vi "get_resolution.vi"(8 "error in (no error)":errorcluster, 11 "TrajectoryDL090201FrameScan in":refnum<class "TrajectoryDL090201FrameScan.lvclass">) -> (0 "error out":errorcluster, 1 "y":i32, 2 "x":i32, 3 "TrajectoryDL090201FrameScan out":refnum<class "TrajectoryDL090201FrameScan.lvclass">)   [LabVIEW 2010, in "TrajectoryDL090201FrameScan.lvclass"]
uses:
  TrajectoryDL090201FrameScan.lvclass
  TrajectoryDL090201FrameScan.lvclass/TrajectoryDL090201FrameScan.ctl
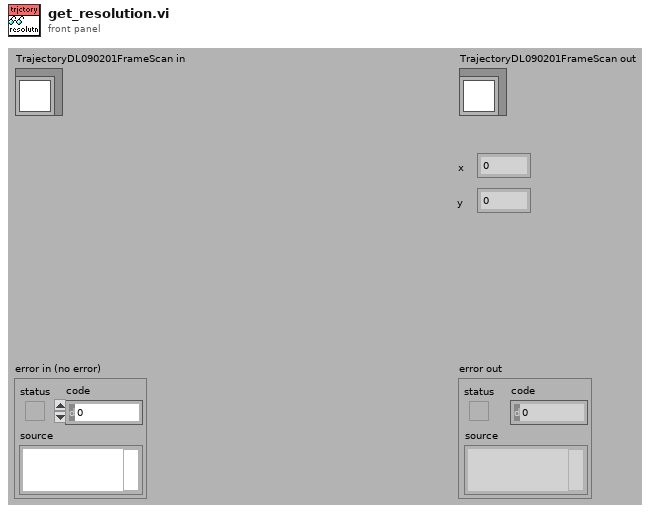
[diagram p1: front panel]
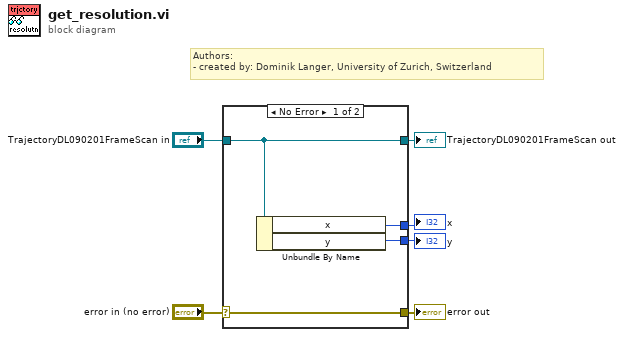
[diagram p0: block diagram]
diagram:
  # "Authors: \n- created by: Dominik Langer, University of Zurich, Switzerland"
  n1 = case shown="No Error" "error in (no error)" {
    selector: "error in (no error)" -> [w10 w11]
    tunnel: [w10 w11] -> w5
    tunnel: [w9 w12] -> w3
    tunnel: "TrajectoryDL090201FrameScan in" -> [w9 w12]
    tunnel: [w8 _] -> w2
    tunnel: [w7 _] -> w1
    frame No Error {
      n2 = Unbundle By Name(w9) -> ("x"=w8:i32, "y"=w7:i32)
    }
    frame Error {
    }
  }
  "error out" <- w5
  "TrajectoryDL090201FrameScan out" <- w3
  "x" <- w2
  "y" <- w1
